vi "SimulatedSensorsGLOBAL (1).vi"() -> ()   [LabVIEW 2017]
panel:
  in  "Temperature (C)":dbl
  in  "Battery Voltage (V)":dbl=27.0
  in  "Simulate Data?":bool
  in  "Sim Distance (m)":dbl
  in  "IMU Temperature (C)":dbl=25.0
  in  "IMU Pressure (Pa)":dbl
  in  "IMU Acceleration (m/s2)":dbl
  in  "Piezo (on/off)":bool
  in  "Acceleration (m/s2)":dbl=0.1
  in  "Linear Pot Voltage (V)":dbl=0.1
  in  "Hall Effect Voltage (V)":dbl=0.1
  in  "Baby Tank Pressure (PSI)":dbl
  in  "Big Tanks Pressure (PSI)":dbl
  in  "Magnetic Brakes Pressure (PSI)":dbl
  in  "Suspension Pressure (PSI)":dbl
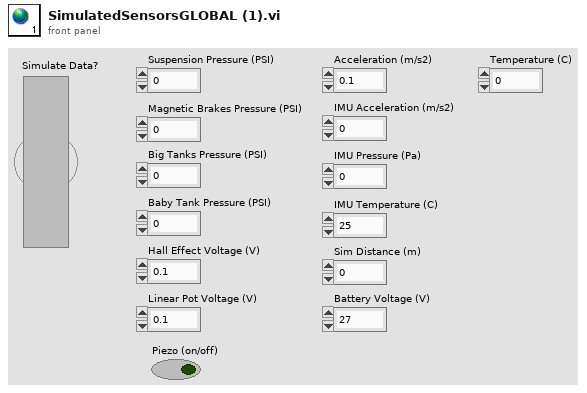
[diagram p1: front panel]
diagram:
